vi "Check GU Selection.vi"(8 "error in":errorcluster, 11 "Curr Cal Cfg":T1) -> (0 "error out":errorcluster, 1 "Info":string, 2 "OK?":bool, 3 "Curr Cal Cfg Out":T1)   [LabVIEW 2020, in "GUCalibration2.lvlib"]
uses:
  GUCalibration2.lvlib
  Controls/Config Data Type.ctl
  Controls/User Facing Msg Enum.ctl
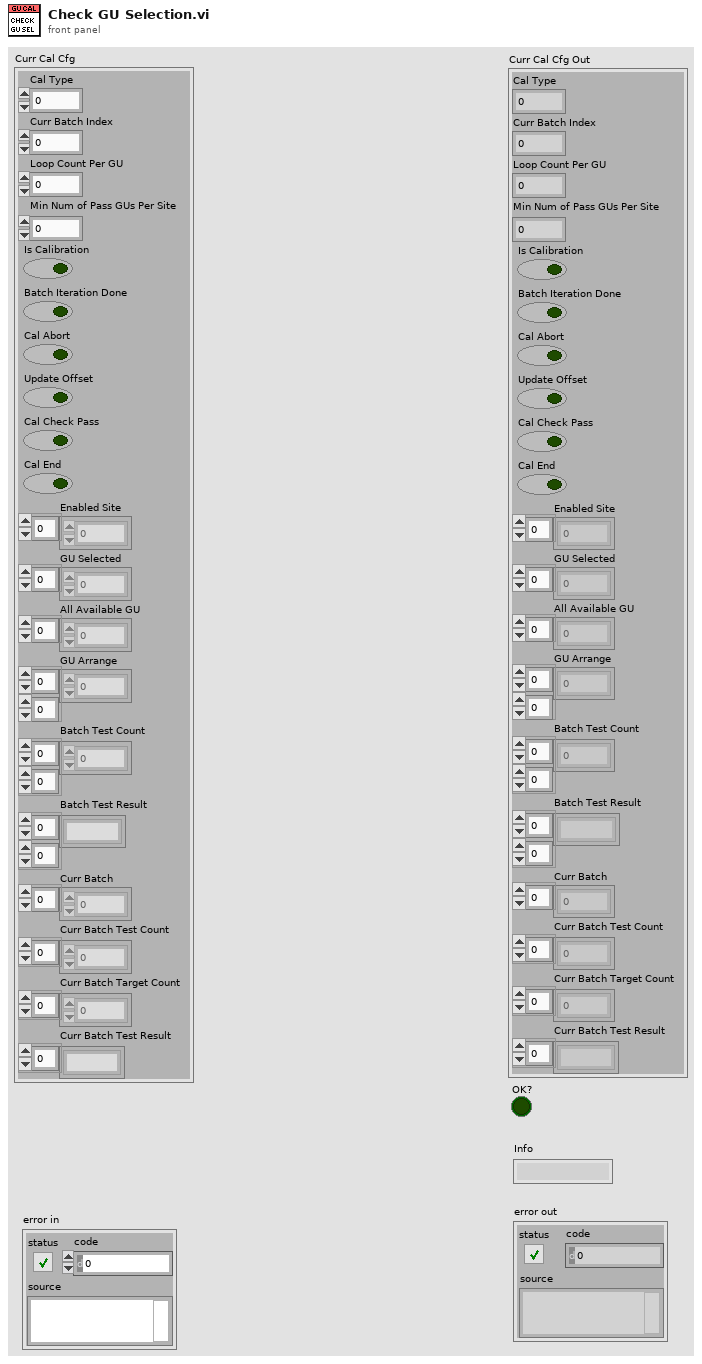
[diagram p1: front panel]
types:
  T1 = typedef "GUCalibration2.lvlib/Config Data Type.ctl" = cluster{"Cal Type":i32, "Curr Batch Index":i32, "Loop Count Per GU":i32, "Min Num of Pass GUs Per Site":i32, "Is Calibration":bool, "Batch Iteration Done":bool, "Cal Abort":bool, "Update Offset":bool, "Cal Check Pass":bool, "Cal End":bool, "Enabled Site":i32[], "GU Selected":i32[], "All Available GU":i32[], "GU Arrange":i32[][], "Batch Test Count":i32[][], "Batch Test Result":string[][], "Curr Batch":i32[], "Curr Batch Test Count":i32[], "Curr Batch Target Count":i32[], "Curr Batch Test Result":string[]}
  T2 = typedef "GUCalibration2.lvlib/User Facing Msg Enum.ctl" = enum16{"Invalid GU Number", "Select More GU", "Exceptional Lot End", "Not All Sites Test", "GU Arrange Error", "Put GU In Sites", "No Cal Site Offset Msg"}
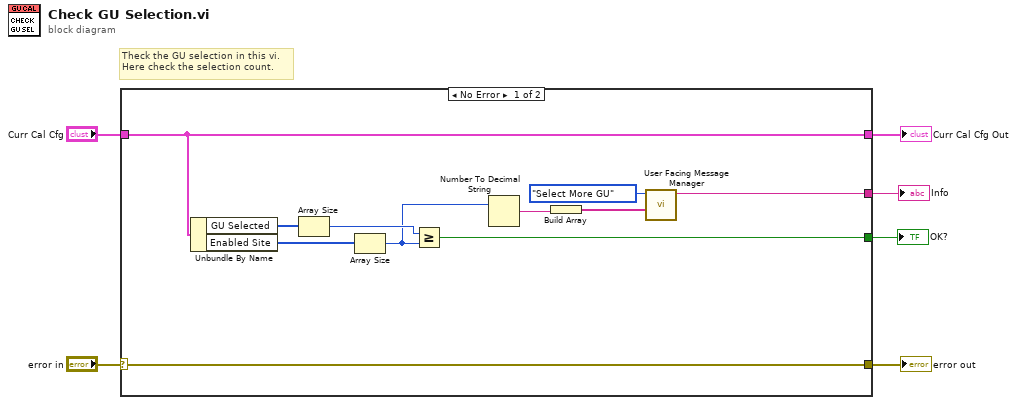
[diagram p0: block diagram]
diagram:
  # "Theck the GU selection in this vi.\nHere check the selection count."
  n1 = case shown="No Error" "error in" {
    selector: "error in" -> [w17 w18]
    tunnel: "Curr Cal Cfg" -> [w14 w19]
    tunnel: [w14 w19] -> w5
    tunnel: [w17 w18] -> w3
    tunnel: [w12 _] -> w2
    tunnel: [w7 _] -> w1
    frame No Error {
      n2 = Unbundle By Name(w14) -> ("GU Selected"=w16:i32[], "Enabled Site"=w15:i32[])
      n3 = Array Size(array=w16) -> (size(s)=w13:i32)
      n4 = Array Size(array=w15) -> (size(s)=w10:i32)
      n5 = Greater Or Equal?(x=w13, y=w10) -> (x >= y?=w12:bool)
      n6 = Number To Decimal String(number=w10) -> (decimal integer string=w9:string)  [unwired: 1 in]
      n7 = Build Array(w9) -> (w8:string[])
      n8 = call "User Facing Message Manager.vi"("Variable Msg"=w8, "User Facing Msg"=User_Facing_Msg_Enum."Select More GU") -> ("User Facing Msg Out"=w7:string)  [unwired: 7 in, 2 out]
    }
    frame Error {
    }
  }
  "Curr Cal Cfg Out" <- w5
  "error out" <- w3
  "OK?" <- w2
  "Info" <- w1
